vi "Idle_WeatherStationCollectionFreqCalc.vi"(8 "Update Period (sec)":i32=5, 10 "Individual Loop Wait Time(ms)":u32=100, 11 "Loop Itteration":i32) -> (3 "Data Collect This Itteration?":bool)   [LabVIEW 2012]
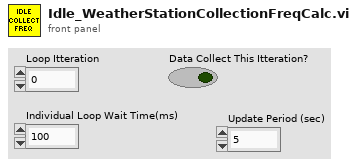
[diagram p1: front panel]
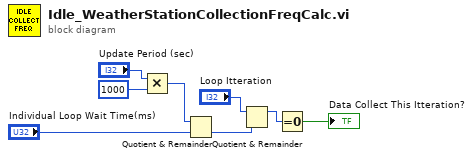
[diagram p0: block diagram]
diagram:
  n1 = Multiply(x="Update Period (sec)", y=1000) -> (x*y=w3:i32)
  n2 = Quotient & Remainder(x=w3, y="Individual Loop Wait Time(ms)") -> (floor(x/y)=w8:u32)  [unwired: 1 out]
  n3 = Quotient & Remainder(x="Loop Itteration", y=w8) -> (x-y*floor(x/y)=w5:u32)  [unwired: 1 out]
  n4 = Equal To 0?(x=w5) -> (x = 0?=→"Data Collect This Itteration?":bool)
